vi "1ship.vi"(11 "Array":u16[][](array[ring])) -> (3 "Array 2":u16[][](array[ring]))   [LabVIEW 2014]
panel:
  in  "Array 20":u16[][](array[ring])=[[1]]
  in  "Raw":i32=1
  in  "Column":i32=1
  in  "?":bool
  out "Boolean":bool
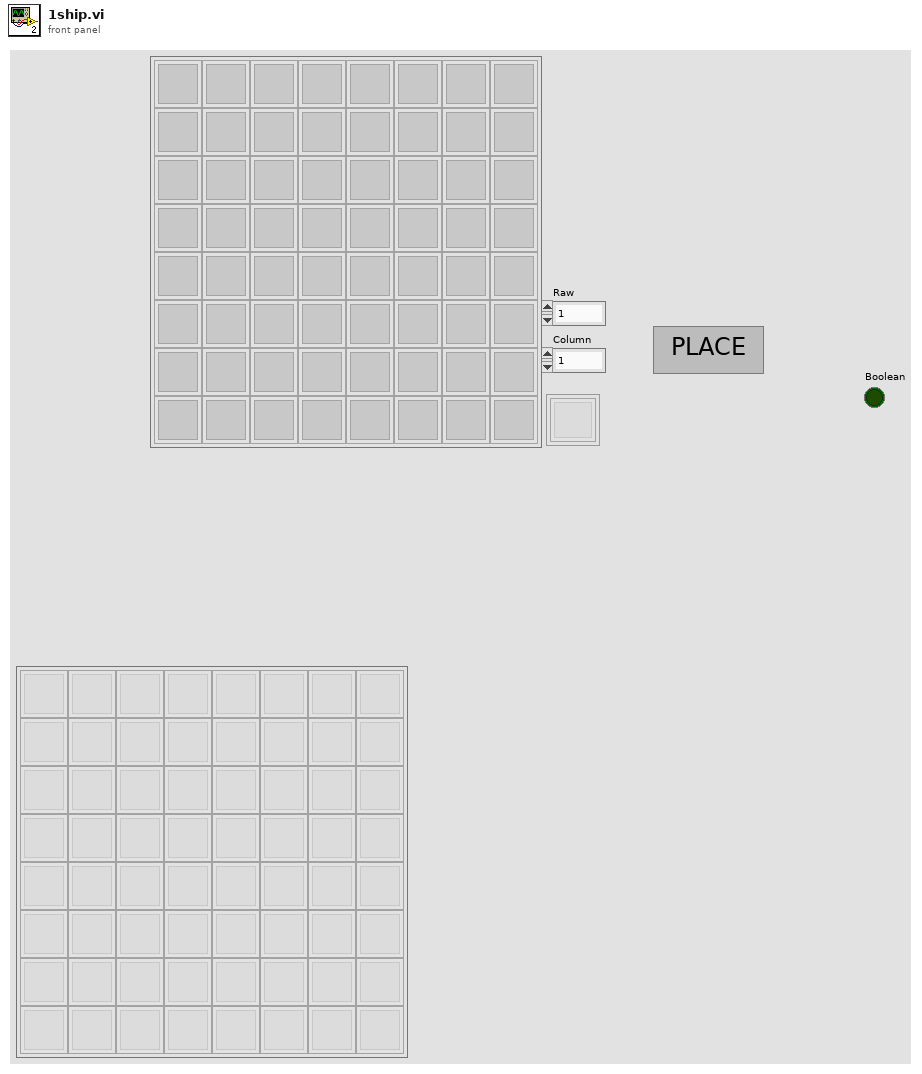
[diagram p1: front panel]
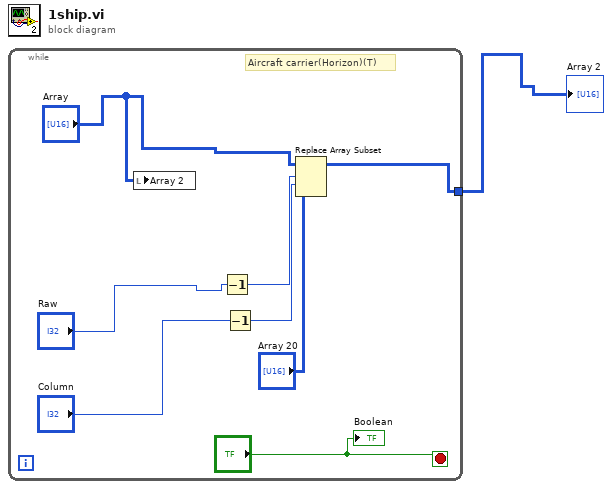
[diagram p0: block diagram]
diagram:
  n1 = while {
    tunnel: [w8] -> w1
    stop <- "?" stop-if-true
    # "Aircraft carrier(Horizon)(T)"
    n2 = local write "Array 2"("Array") -> ()
    n3 = Decrement(x="Raw") -> (x-1=w6:i32)
    n4 = Decrement(x="Column") -> (x-1=w4:i32)
    n5 = Replace Array Subset(array="Array", new element="Array 20", index (row)=w6, index (col)=w4) -> (w8:u16[][])
    "Boolean" <- "?"
  }
  "Array 2" <- w1
